vi "Get Object Parameter - Object.vi"(8 "error in (no error)":errorcluster, 10 "Parameter Name":string, 11 "JSON Tree In (JSON Object)":variant) -> (0 "error out":errorcluster, 1 "is JSON Null?":bool, 2 "JSON Object":variant, 3 "JSON Tree Out Passthrough":variant)   [LabVIEW 2013, in "i3-json.lvlib"]
doc: "Use this template to build a VI to use as a subVI."
uses:
  i3-json.lvlib
  JSON Types/JSON Type.ctl
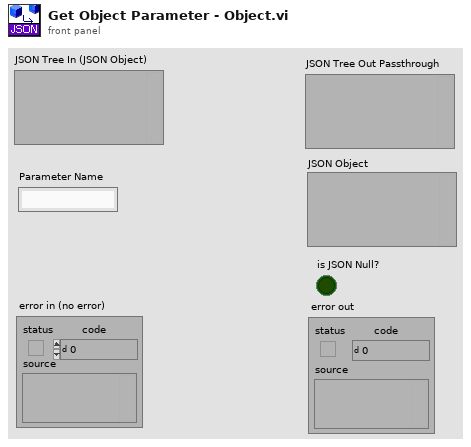
[diagram p1: front panel]
types:
  T1 = typedef "i3-json.lvlib/JSON Type.ctl" = enum8{"JSON Compatible", "JSON Array", "JSON Object", "JSON Null", "Double", "String", "Boolean", "Unknown", "Data JSON string"}
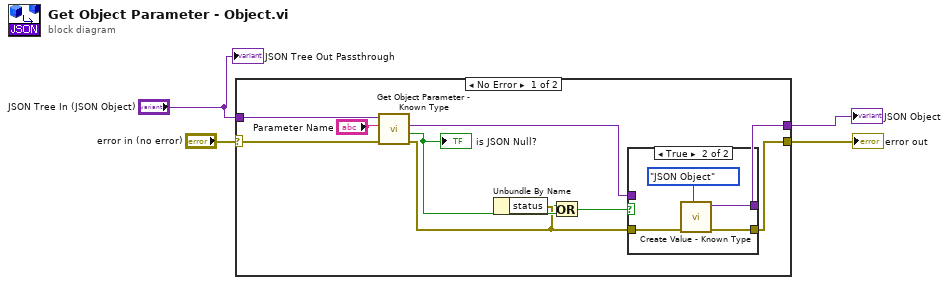
[diagram p0: block diagram]
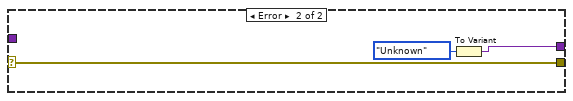
[diagram p3: hidden frame]
diagram:
  n1 = case shown="No Error" "error in (no error)" {
    selector: "error in (no error)" -> [w13 w23]
    tunnel: [w11 w23] -> w3
    tunnel: "JSON Tree In (JSON Object)" -> [w14 _]
    tunnel: [w9 w21] -> w2
    frame No Error {
      n2 = call "Get Object Parameter - Known Type.vi"("error in (no error)"=w13, "Parameter Name"="Parameter Name", "JSON Tree In (JSON Object)"=w14) -> ("error out"=w6:errorcluster, "is JSON Null?"=w8:bool, "Value"=w10:variant)  [unwired: 3 in, 3 out]
      "is JSON Null?" <- w8
      n3 = Unbundle By Name(w6) -> ("status"=w5:bool)
      n4 = Or(x=w5, y=w8) -> (x .or. y?=w12:bool)
      n5 = case shown="True" w12 {
        tunnel: w6 -> [w15 w19]
        tunnel: [w15 w18] -> w11
        tunnel: w10 -> [w16 _]
        tunnel: [w16 w17] -> w9
        frame False {
        }
        frame True {
          n6 = call "Create Value - Known Type.vi"("JSON Type"=JSON_Type."JSON Object", "error in (no error)"=w19) -> ("error out"=w18:errorcluster, "JSON Tree"=w17:variant)  [unwired: 8 in]
        }
      }
    }
    frame Error {
      n7 = To Variant(anything=JSON_Type."Unknown" ("JSON Type")) -> (Variant=w21:variant)
    }
  }
  "error out" <- w3
  "JSON Object" <- w2
  "JSON Tree Out Passthrough" <- "JSON Tree In (JSON Object)"
